vi "Temp ctrl - Ramp Setpoint.vi"(8 "Error In":errorcluster, 9 "Speed":dbl[unit], 10 "Setpoint":dbl[unit], 11 "Temp handle":T1={"Connected"=FALSE, "Temp ctrl"={"Gain (P)"=0.0, "Reset (I)"=0.0, "Rate (D)"=0, "Stabilization rate"=0.0, "Stabilization delta"=0.0, "Type"=enum."Lake Shore 325", "Custom temp ctrl"={"VISA resource name"=""}, "Lakeshore 325"={"VISA name"="", "Loop"=0, "Heater Range"=1, "Heater Resistance"=0, "Sample sensor"=0, "Fast sensor"=0, "Slow sensor"=0}}} {"Temp ctrl"."Lakeshore 325"."Slow sensor" items=["A", "B"]; "Temp ctrl"."Lakeshore 325"."Fast sensor" items=["A", "B"]; "Temp ctrl"."Lakeshore 325"."Sample sensor" items=["A", "B"]; "Temp ctrl"."Lakeshore 325"."Heater Resistance" items=["25 Ohm"=1, "50 Ohm"=2]; "Temp ctrl"."Lakeshore 325"."Heater Range" items=["Off", "Low (loop 1) or On (loop 2)", "High (loop 1)"]; "Temp ctrl"."Lakeshore 325"."Loop" items=["Loop 1"=1, "Loop 2"=2]}) -> (0 "Error Out":errorcluster)   [LabVIEW 2019]
doc: "Applies temperature controller setpoint in a ramp mode"
uses:
  Type defs/Temp handle Type Def.ctl
  Type defs/Temp ctrl Type Def.ctl
  Custom devices/Custom temp ctrl settings.ctl
  <instrlib>/Lake Shore 325/Lake Shore 325.lvlib
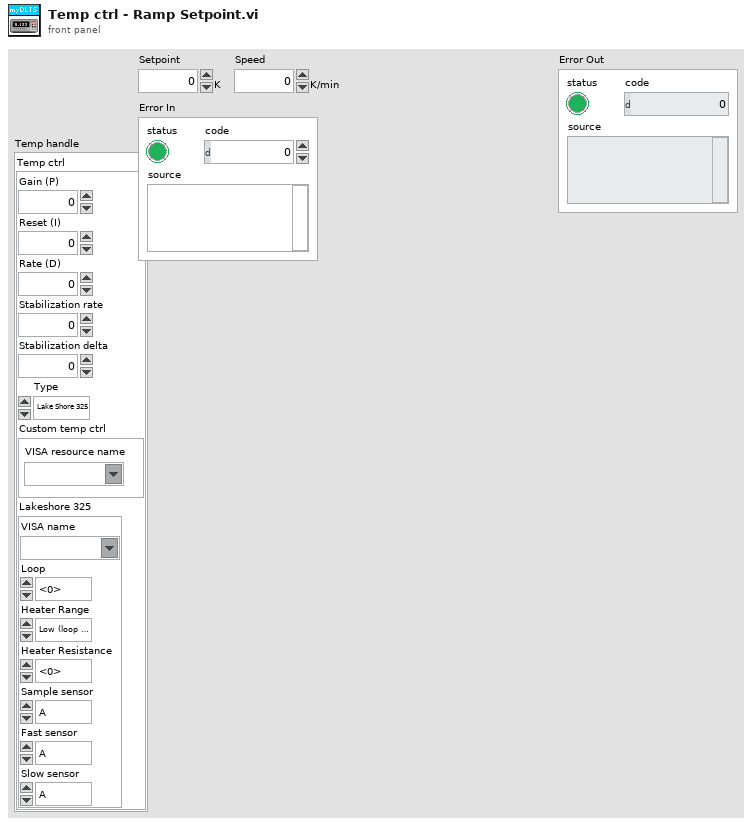
[diagram p1: front panel]
types:
  T1 = typedef "Temp handle Type Def.ctl" = cluster{"Connected":bool, "Temp ctrl":T2}
  T2 = typedef "Temp ctrl Type Def.ctl" = cluster{"Gain (P)":dbl, "Reset (I)":dbl, "Rate (D)":u16, "Stabilization rate":dbl, "Stabilization delta":dbl, "Type":enum16{"Custom", "Lake Shore 325"}, "Custom temp ctrl":T3, "Lakeshore 325":cluster{"VISA name":refnum<visa-resource-name>, "Loop":u16, "Heater Range":u16, "Heater Resistance":u16, "Sample sensor":u16, "Fast sensor":u16, "Slow sensor":u16}}
  T3 = typedef "Custom temp ctrl settings.ctl" = cluster{"VISA resource name":refnum<visa-resource-name>}
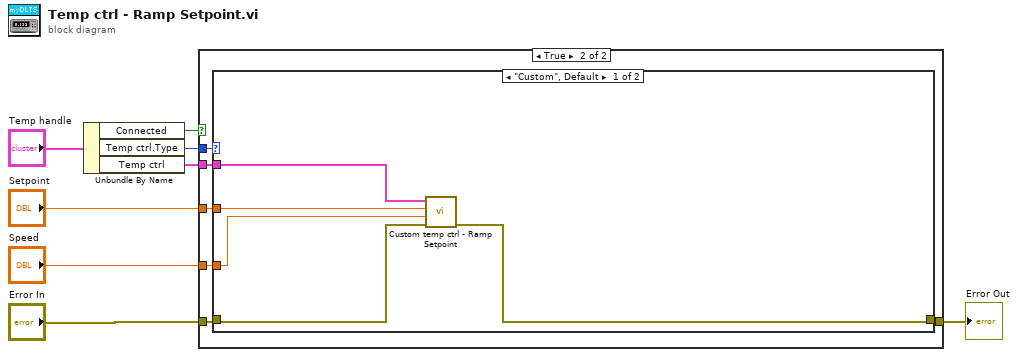
[diagram p0: block diagram]
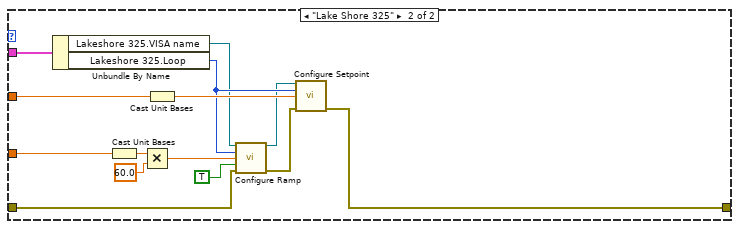
[diagram p3: hidden frame]
diagram:
  n1 = Unbundle By Name("Temp handle") -> ("Connected"=w8:bool, "Temp ctrl.Type"=w7:enum16{"Custom", "Lake Shore 325"}, "Temp ctrl"=w5:T2)
  n2 = case shown="True" w8 {
    tunnel: w7 -> [_ w15]
    tunnel: w5 -> [_ w14]
    tunnel: "Setpoint" -> [_ w13]
    tunnel: "Error In" -> [w9 w12]
    tunnel: [w9 w11] -> w2
    tunnel: "Speed" -> [_ w10]
    frame False {
    }
    frame True {
      n3 = case shown="\"Custom\", Default" w15 {
        tunnel: w14 -> [w18 w34]
        tunnel: w13 -> [w17 w33]
        tunnel: w12 -> [w20 w29]
        tunnel: [w19 w31] -> w11
        tunnel: w10 -> [w16 w30]
        frame "Custom", Default {
          n4 = call "Custom temp ctrl - Ramp Setpoint.vi"("Error In"=w20, "Speed"=w16, "Setpoint"=w17, "Temp ctrl"=w18) -> ("Error Out"=w19:errorcluster)  [unwired: 7 in]
        }
        frame "Lake Shore 325" {
          n5 = Unbundle By Name(w34) -> ("Lakeshore 325.VISA name"=w27:refnum<visa-resource-name>, "Lakeshore 325.Loop"=w28:u16)
          n6 = Cast Unit Bases(0:w30) -> (2:w22:dbl)  [unwired: 1 in]
          n7 = Multiply(x=w22, y=60.0) -> (x*y=w21:dbl)
          n8 = Cast Unit Bases(0:w33) -> (2:w32:dbl)  [unwired: 1 in]
          n9 = call <instrlib>:"Configure Ramp.vi"("VISA resource name"=w27, "Loop (1:Loop 1)"=w28, "Rate Value (0.0)"=w21, "Setpoint Ramp (F: Off)"=TRUE, "error in (no error)"=w29) -> ("VISA resource name out"=w26:refnum<visa-resource-name>, "error out"=w25:errorcluster)  [unwired: 9 in]
          n10 = call <instrlib>:"Configure Setpoint.vi"("VISA resource name"=w26, "Loop (1:Loop 1)"=w28, "Setpoint Value (0.0000)"=w32, "error in (no error)"=w25) -> ("error out"=w31:errorcluster)  [unwired: 10 in, 1 out]
        }
      }
    }
  }
  "Error Out" <- w2
